vi "SimpleAnyBuilder.vi"() -> ()   [LabVIEW 2019]
uses:
  labview source/gRPC lv Support/Shared/Any.ctl
  labview source/gRPC lv Support/Server API/typeDefs/Message Metadata.ctl
  labview source/gRPC lv Support/Server API/typeDefs/Message Element Metadata.ctl
  labview source/gRPC lv Support/Server API/typeDefs/Message Element Type.ctl
  50cd6ca9-b915-40c5-a5da-5a0bdd109e0e.vi
  f62721b2-a209-4c6b-affd-5652a03b42cf.vi
  65d46b58-227a-49f8-b739-8ba8c807fa65.vi
  labview source/gRPC lv Support/Server API/Translate Protobuf Error.vi
  <vilib>/AdvancedString/1D String Array to Delimited String.vi
  labview source/gRPC lv Support/Server API/Server/Get Server DLL Path.vi
  labview source/gRPC lv Support/grpc-lvsupport.lvlib
panel:
  out "error out":errorcluster
  out "Numeric 2":i32
  out "Any":T1
  out "Numeric":i32
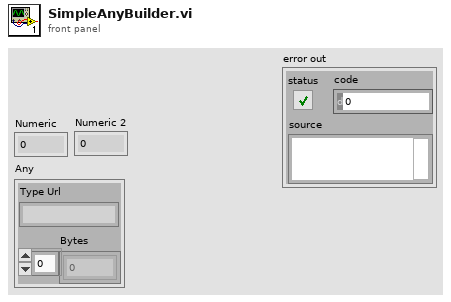
[diagram p1: front panel]
types:
  T1 = typedef "grpc-lvsupport.lvlib/Any.ctl" = cluster{"Type Url":string, "Bytes":u8[]}
  T2 = typedef "grpc-lvsupport.lvlib/Message Element Type.ctl" = enum32{"Int32Value", "FloatValue", "DoubleValue", "BoolValue", "StringValue", "MessageValue", "Int64Value", "UInt32Value", "UInt64Value", "EnumValue", "Bytes", "Fixed64", "Fixed32", "SFixed64", "SFixed32", "SInt64", "SInt32"}
  T3 = typedef "grpc-lvsupport.lvlib/Message Metadata.ctl" = cluster{"Version":i32, "Name":string, "Type Url":string, "Elements":T4[]}
  T4 = typedef "grpc-lvsupport.lvlib/Message Element Metadata.ctl" = cluster{"Embedded Message Name":string, "Protobuf Index":i32, "MessageElementType":T2, "Repeated":bool}
  T5 = typedef "grpc-lvsupport.lvlib/grpcId.ctl" = u64
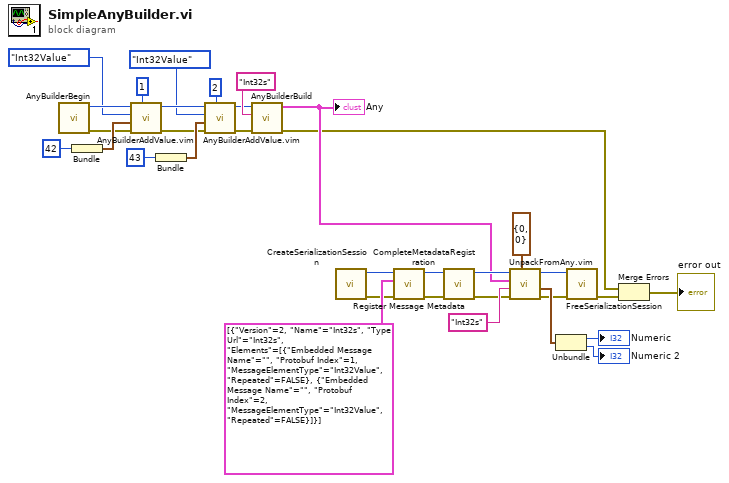
[diagram p0: block diagram]
diagram:
  n1 = call "AnyBuilderBegin.vi"() -> ("error out"=w10:errorcluster, "Builder Ref Out"=w33:T5)  [unwired: 9 in]
  n2 = Bundle(42) -> (w30:cluster{i32})  [unwired: 1 in]
  n3 = call "AnyBuilderAddValue.vim"("protobufId"=1, "error in"=w10, "Value"=w30, "MessageElementType"=Message_Element_Type."Int32Value", "gRPCid in"=w33) -> ("error out"=w9:errorcluster, "gRPCid out"=w17:u64)  [unwired: 5 in]
  n4 = Bundle(43) -> (w13:cluster{i32})  [unwired: 1 in]
  n5 = call "AnyBuilderAddValue.vim"("protobufId"=2, "error in"=w9, "Value"=w13, "MessageElementType"=Message_Element_Type."Int32Value", "gRPCid in"=w17) -> ("error out"=w8:errorcluster, "gRPCid out"=w11:u64)  [unwired: 5 in]
  n6 = call "AnyBuilderBuild.vi"("error in"=w8, "Message Type"="Int32s", "Builder Ref"=w11) -> ("error out"=w3:errorcluster, "Any"=w23:T1)  [unwired: 7 in]
  "Any" <- w23
  n7 = call "CreateSerializationSession.vi"() -> ("error out"=w7:errorcluster, "Serialization Session ID"=w28:T5)  [unwired: 10 in]
  n8 = call "Register Message Metadata.vi"("error in"=w7, "Messages"=T3[] [{"Version"=2, "Name"="Int32s", "Type Url"="Int32s", "Elements"=[{"Embedded Message Name"="", "Protobuf Index"=1, "MessageElementType"=enum."Int32Value", "Repeated"=FALSE}, {"Embedded Message Name"="", "Protobuf Index"=2, "MessageElementType"=enum."Int32Value", "Repeated"=FALSE}]}], "gRPCid in"=w28) -> ("error out"=w6:errorcluster, "gRPCid out"=w25:T5)  [unwired: 7 in]
  n9 = call "CompleteMetadataRegistration.vi"("error in"=w6, "gRPC ID in"=w25) -> ("error out"=w5:errorcluster, "gRPC ID Out"=w24:T5)  [unwired: 8 in]
  n10 = call "UnpackFromAny.vim"("Data Type"=cluster{i32, i32} {0, 0}, "error in"=w5, "Message Type"="Int32s", "Any"=w23, "gRPCid in"=w24) -> ("error out"=w4:errorcluster, "Unpacked Value"=w20:cluster{i32, i32}, "gRPCid out"=w18:u64)  [unwired: 4 in]
  n11 = Unbundle(w20) -> (→"Numeric":i32, →"Numeric 2":i32)
  n12 = call "FreeSerializationSession.vi"("error in"=w4, "Serialization Session ID"=w18) -> ("error out"=w2:errorcluster)  [unwired: 9 in]
  n13 = Merge Errors(w3, w2) -> (→"error out":errorcluster)
